vi "Add Msg To Seq.vi"(8 "error in (no error)":errorcluster, 10 "Message Name":string, 11 "ICD System Tree View in":refnum<class "[V]System Tree View.lvclass">) -> (0 "error out":errorcluster, 3 "ICD System Tree View out":refnum<class "[V]System Tree View.lvclass">)   [LabVIEW 2020]
uses:
  [V]System Tree View.lvclass
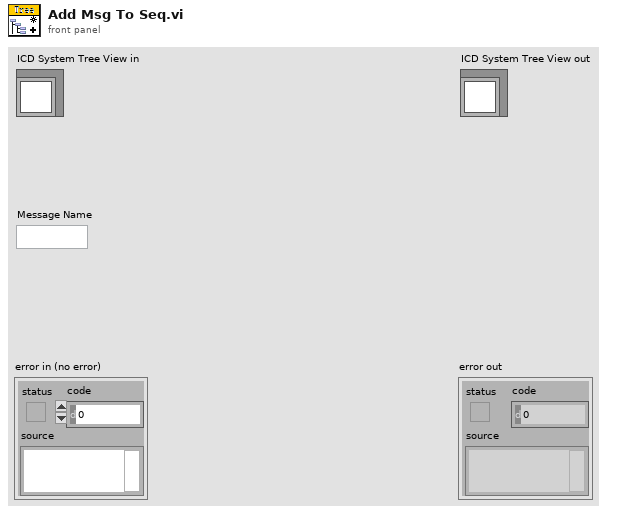
[diagram p1: front panel]
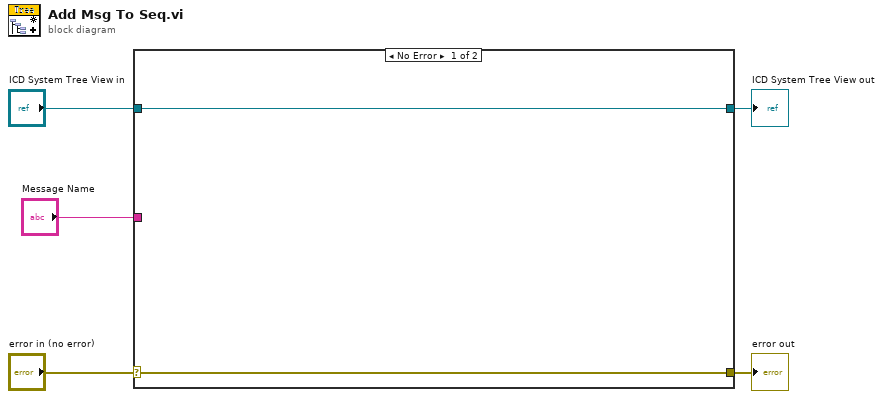
[diagram p0: block diagram]
diagram:
  n1 = case shown="No Error" "error in (no error)" {
    selector: "error in (no error)" -> [w6 w9]
    tunnel: [w6 w9] -> w4
    tunnel: [w7 w8] -> w2
    tunnel: "ICD System Tree View in" -> [w7 w8]
    tunnel: "Message Name" -> [_ _]
    frame No Error {
    }
    frame Error {
    }
  }
  "error out" <- w4
  "ICD System Tree View out" <- w2
